vi "CRYResize Panel Current.vi"(6 "Bar_shadow":refnum<vi>, 7 "DataView Array Idx":i32, 8 "close_panel":bool=TRUE, 9 "spliter array":refnum<vi>[](array[refnum]), 10 "SubPanel array":refnum<vi>[](array[refnum])) -> ()   [LabVIEW 2013]
uses:
  CRYNew View Global.vi
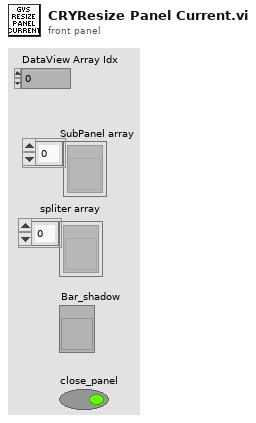
[diagram p1: front panel]
types:
  T1 = typedef "Graph Main Info Cluster.ctl" = cluster{"Selected_BarIdx":i32, "Selected_PanelIdx":i32, "Graph Main VIRef":refnum<vi>, "ToolBarClick":bool, "Spliter Ref Array":refnum<vi>[], "Panel Ref Array":refnum<vi>[], "Spliter_matrix":i32[][], "Panel_matrix":i32[][], "child_spliterIdx_matrix":i32[][], "split_pos_matrix":i32[][], "Title State":bool, "sQueueName":string, "Frame nID":i32, "Graph VIRef Array":cluster{"Graph VIRef":refnum<vi>, "Panel Idx":i32, "Frame VIRef":refnum<vi>, "Icon Ring":i32, "Graph Type":string}[], "View Type":string}
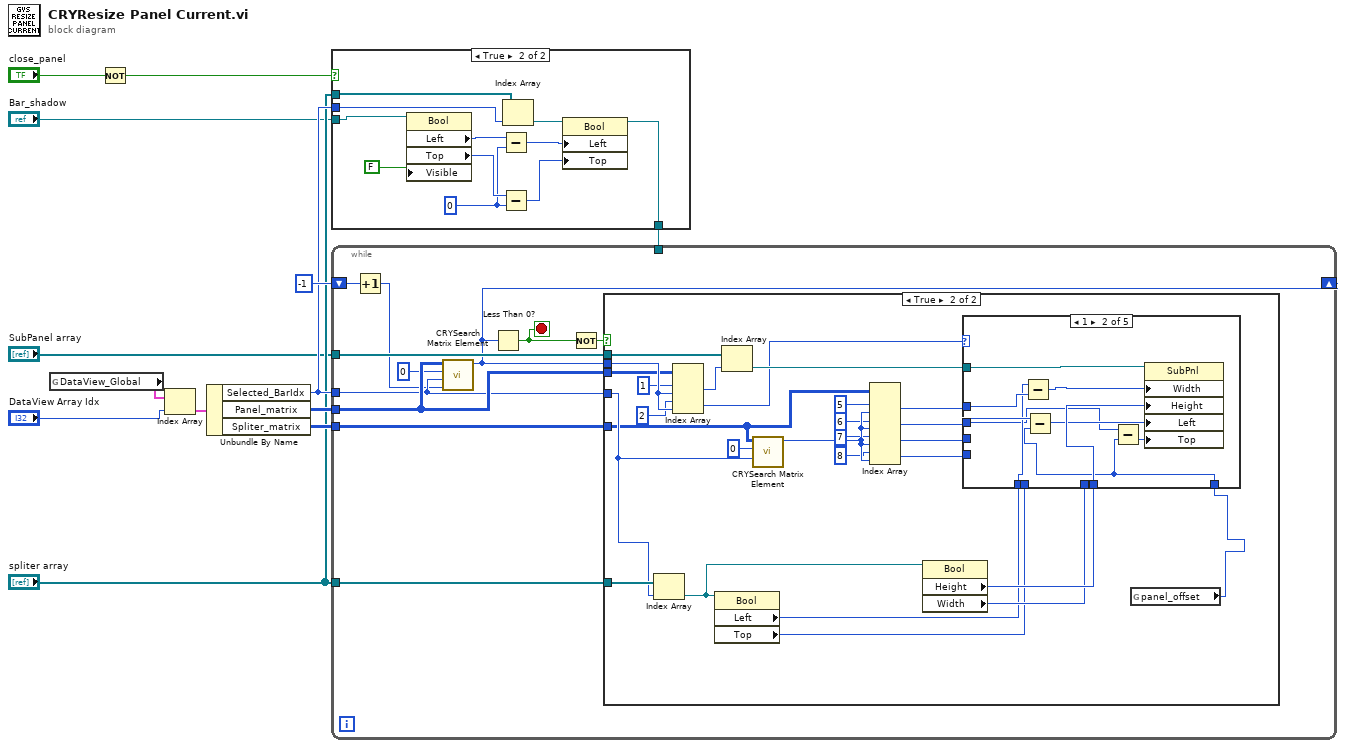
[diagram p0: block diagram]
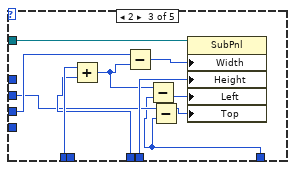
[diagram p5: hidden frame]
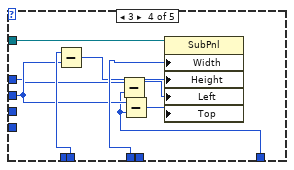
[diagram p6: hidden frame]
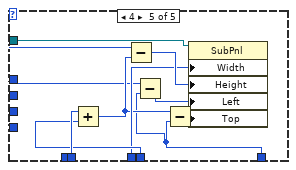
[diagram p7: hidden frame]
diagram:
  n1 = global read "CRYNew View Global.vi" "DataView_Global"() -> (w4:T1[])
  n2 = Not(x="close_panel") -> (.not. x?=w6:bool)
  n3 = Index Array(array=w4, index="DataView Array Idx") -> (element=w5:T1)
  n4 = Unbundle By Name(w5) -> ("Selected_BarIdx"=w12:i32, "Panel_matrix"=w11:i32[][], "Spliter_matrix"=w10:i32[][])
  n5 = case shown="True" w6 {
    tunnel: "spliter array" -> [_ w24]
    tunnel: w12 -> [_ w23]
    tunnel: "Bar_shadow" -> [_ w15]
    tunnel: [_ w14] -> w1
    frame False {
    }
    frame True {
      w16 = 0 ("y")
      n6 = property class="Bool"(reference=w15, "Visible"=FALSE) -> ("Left"=w20:i32, "Top"=w18:i32)  [unwired: 1 in, 2 out]
      n7 = Subtract(x=w20, y=w16) -> (x-y=w19:i32)
      n8 = Subtract(x=w18, y=w16) -> (x-y=w17:i32)
      n9 = Index Array(array=w24, index=w23) -> (element=w22:refnum<vi>)
      n10 = property class="Bool"(reference=w22, "Left"=w19, "Top"=w17) -> (reference out=w14:refnum<vi>)  [unwired: 1 in, 1 out]
    }
  }
  n11 = while {
    shift-right: [w27] -> _
    shift-left: -1 -> [w26]
    tunnel: w12 -> [w30]
    tunnel: "SubPanel array" -> [w35]
    tunnel: "spliter array" -> [w25]
    tunnel: w11 -> [w31]
    tunnel: w10 -> [w32]
    tunnel: w1 -> [_]
    stop <- w34 stop-if-true
    n12 = Increment(x=w26) -> (x+1=w28:i32)
    n13 = call "CRYSearch Matrix Element.vi"("start index"=w28, "element"=w30, "index (row)"=0, "matrix in"=w31) -> ("index of element"=w27:i32)  [unwired: 7 in]
    n14 = Less Than 0?(x=w27) -> (x < 0?=w34:bool)
    n15 = Not(x=w34) -> (.not. x?=w33:bool)
    n16 = case shown="True" w33 {
      tunnel: w27 -> [_ w47]
      tunnel: w35 -> [_ w61]
      tunnel: w25 -> [_ w62]
      tunnel: w30 -> [_ w59]
      tunnel: w31 -> [_ w46]
      tunnel: w32 -> [_ w57]
      frame False {
      }
      frame True {
        n17 = Index Array(array=w62, index=w59) -> (element=w39:refnum<vi>)
        n18 = Index Array(array=w46, index (row) #1=1 ("index (row)"), index (col) #1=w47, index (row) #2=2 ("index (row)"), index (col) #2=w47) -> (element #1=w43:i32, element #2=w42:i32)
        n19 = property class="Bool"(reference=w39) -> ("Left"=w38:i32, "Top"=w37:i32)  [unwired: 1 in, 2 out]
        n20 = Index Array(array=w61, index=w43) -> (element=w60:refnum<vi>)
        n21 = call "CRYSearch Matrix Element.vi"("element"=w59, "index (row)"=0, "matrix in"=w57) -> ("index of element"=w56:i32)  [unwired: 8 in]
        n22 = Index Array(array=w57, index (row) #1=5 ("index (row)"), index (col) #1=w56, index (row) #2=6 ("index (row)"), index (col) #2=w56, index (row) #3=7 ("index (row)"), index (col) #3=w56, index (row) #4=8 ("index (row)"), index (col) #4=w56) -> (element #1=w51:i32, element #2=w50:i32, element #3=w49:i32, element #4=w48:i32)
        n23 = property class="Bool"(reference=w39) -> ("Height"=w41:u32, "Width"=w40:u32)  [unwired: 1 in, 2 out]
        n24 = global read "CRYNew View Global.vi" "panel_offset"() -> (w36:i32)
        n25 = case shown="1" w42 {
          tunnel: w51 -> [_ w71 _ w85 w94]
          tunnel: w50 -> [_ w64 w74 w86 _]
          tunnel: w49 -> [_ _ w81 _ _]
          tunnel: w48 -> [_ _ _ _ w101]
          tunnel: w60 -> [_ w70 w82 w91 w102]
          tunnel: w38 -> [_ w69 w78 _ _]
          tunnel: w37 -> [_ _ _ w89 w99]
          tunnel: w41 -> [_ w68 w79 _ w98]
          tunnel: w40 -> [_ _ w77 w90 w97]
          tunnel: w36 -> [_ w63 w72 w83 w92]
          frame 0, Default {
          }
          frame 1 {
            n26 = Subtract(x=w69, y=w71) -> (x-y=w67:i32)
            n27 = Subtract(x=w71, y=w63) -> (x-y=w66:i32)
            n28 = Subtract(x=w64, y=w63) -> (x-y=w65:i32)
            n29 = property class="SubPnl"(reference=w70, "Width"=w67, "Height"=w68, "Left"=w66, "Top"=w65) -> ()  [unwired: 1 in, 2 out]
          }
          frame 2 {
            n30 = Add(x=w78, y=w77) -> (x+y=w76:u32)
            n31 = Subtract(x=w81, y=w76) -> (x-y=w80:u32)
            n32 = Subtract(x=w76, y=w72) -> (x-y=w75:u32)
            n33 = Subtract(x=w74, y=w72) -> (x-y=w73:i32)
            n34 = property class="SubPnl"(reference=w82, "Width"=w80, "Height"=w79, "Left"=w75, "Top"=w73) -> ()  [unwired: 1 in, 2 out]
          }
          frame 3 {
            n35 = Subtract(x=w89, y=w86) -> (x-y=w88:i32)
            n36 = Subtract(x=w85, y=w83) -> (x-y=w84:i32)
            n37 = Subtract(x=w86, y=w83) -> (x-y=w87:i32)
            n38 = property class="SubPnl"(reference=w91, "Width"=w90, "Height"=w88, "Left"=w84, "Top"=w87) -> ()  [unwired: 1 in, 2 out]
          }
          frame 4 {
            n39 = Add(x=w99, y=w98) -> (x+y=w96:u32)
            n40 = Subtract(x=w101, y=w96) -> (x-y=w100:u32)
            n41 = Subtract(x=w94, y=w92) -> (x-y=w93:i32)
            n42 = Subtract(x=w96, y=w92) -> (x-y=w95:u32)
            n43 = property class="SubPnl"(reference=w102, "Width"=w97, "Height"=w100, "Left"=w93, "Top"=w95) -> ()  [unwired: 1 in, 2 out]
          }
        }
      }
    }
  }
